vi "v2.61.vi"() -> ()   [LabVIEW 2018]
uses:
  <vilib>/DAQmx/read.llb/DAQmx Read (Analog 1D DBL NChan 1Samp).vi
  <extravilib>/ChannelInstances/High Speed Stream-c(a[.](c(dbl,dbl,dbl,dbl)),stamp,a[.](dbl),c(dbl,dbl,dbl,dbl,dbl,dbl,dbl))/_Read For Replicate.vi
  <extravilib>/ChannelInstances/High Speed Stream-c(a[.](c(dbl,dbl,dbl,dbl)),stamp,a[.](dbl),c(dbl,dbl,dbl,dbl,dbl,dbl,dbl))/Instantiate.vi
  <vilib>/Utility/file.llb/Write Delimited Spreadsheet (string).vi
  <extravilib>/ChannelInstances/High Speed Stream-c(a[.](c(dbl,dbl,dbl,dbl)),stamp,a[.](dbl),c(dbl,dbl,dbl,dbl,dbl,dbl,dbl))/)Channel.vi
  <extravilib>/ChannelInstances/High Speed Stream-c(a[.](c(dbl,dbl,dbl,dbl)),stamp,a[.](dbl),c(dbl,dbl,dbl,dbl,dbl,dbl,dbl))/Abort Signal/Init Signal.vi
  <vilib>/DAQmx/create/channels.llb/DAQmx Create Channel (AI-Temperature-Thermocouple).vi
  <vilib>/DAQmx/configure/timing.llb/DAQmx Timing (Sample Clock).vi
  <vilib>/DAQmx/miscellaneous.llb/DAQmx Fill In Error Info.vi
  <extravilib>/ChannelInstances/High Speed Stream-c(a[.](c(dbl,dbl,dbl,dbl)),stamp,a[.](dbl),c(dbl,dbl,dbl,dbl,dbl,dbl,dbl)).lvlib
panel:
  in  "file path (dialog if empty)":path
  out "Enum":T1(ring)
  in  "Start Recording?":bool
  in  "Stop Recording?":bool
  in  "Flowrate Control":dbl
  out "Status":T2(ring)
  in  "OK Button":bool
  in  "DAQ Properties":cluster{"Sample Rate":dbl}={"Sample Rate"=1.0} {"Sample Rate" min=1.0 max=10000.0 step=1.0}
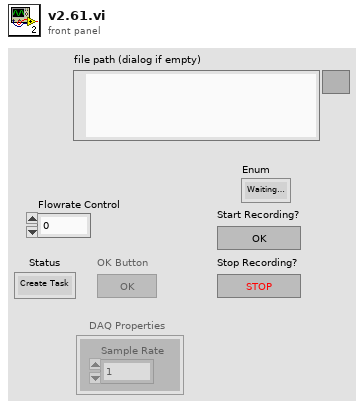
[diagram p1: front panel]
types:
  T1 = enum16{"Waiting to record", "Creating Spreadsheet", "Recording", "Finished Recording"}
  T2 = enum16{"Create Task", "Change Settings", "Check Settings", "Read Data", "End Task"}
  T3 = enum8{"Enabled", "Disabled", "Disabled and Grayed Out"}
  T4 = cluster{"Flowrate Data":cluster{"Line Number":dbl, "Temperature":dbl, "Pressure":dbl, "Flowrate":dbl}[], "Current Time":timestamp, "DAQmx Data":dbl[], "Rig Temperatures":cluster{"BRNR FC":dbl, "BRNR Nozzle":dbl, "Lance Tip":dbl, "Tube 2 Tmp":dbl, "Tube Tmp":dbl, "GA GAS Tmp":dbl, "Chamber External Temp":dbl}}
  T5 = cluster{"BRNR FC":dbl, "BRNR Nozzle":dbl, "Lance Tip":dbl, "Tube 2 Tmp":dbl, "Tube Tmp":dbl, "GA GAS Tmp":dbl, "Chamber External Temp":dbl}
  T6 = cluster{"Line Number":dbl, "Temperature":dbl, "Pressure":dbl, "Flowrate":dbl}[]
  T7 = typedef "High Speed Stream-c(a[.](c(dbl,dbl,dbl,dbl)),stamp,a[.](dbl),c(dbl,dbl,dbl,dbl,dbl,dbl,dbl)).lvlib/)Channel.ctl" = refnum<queue>
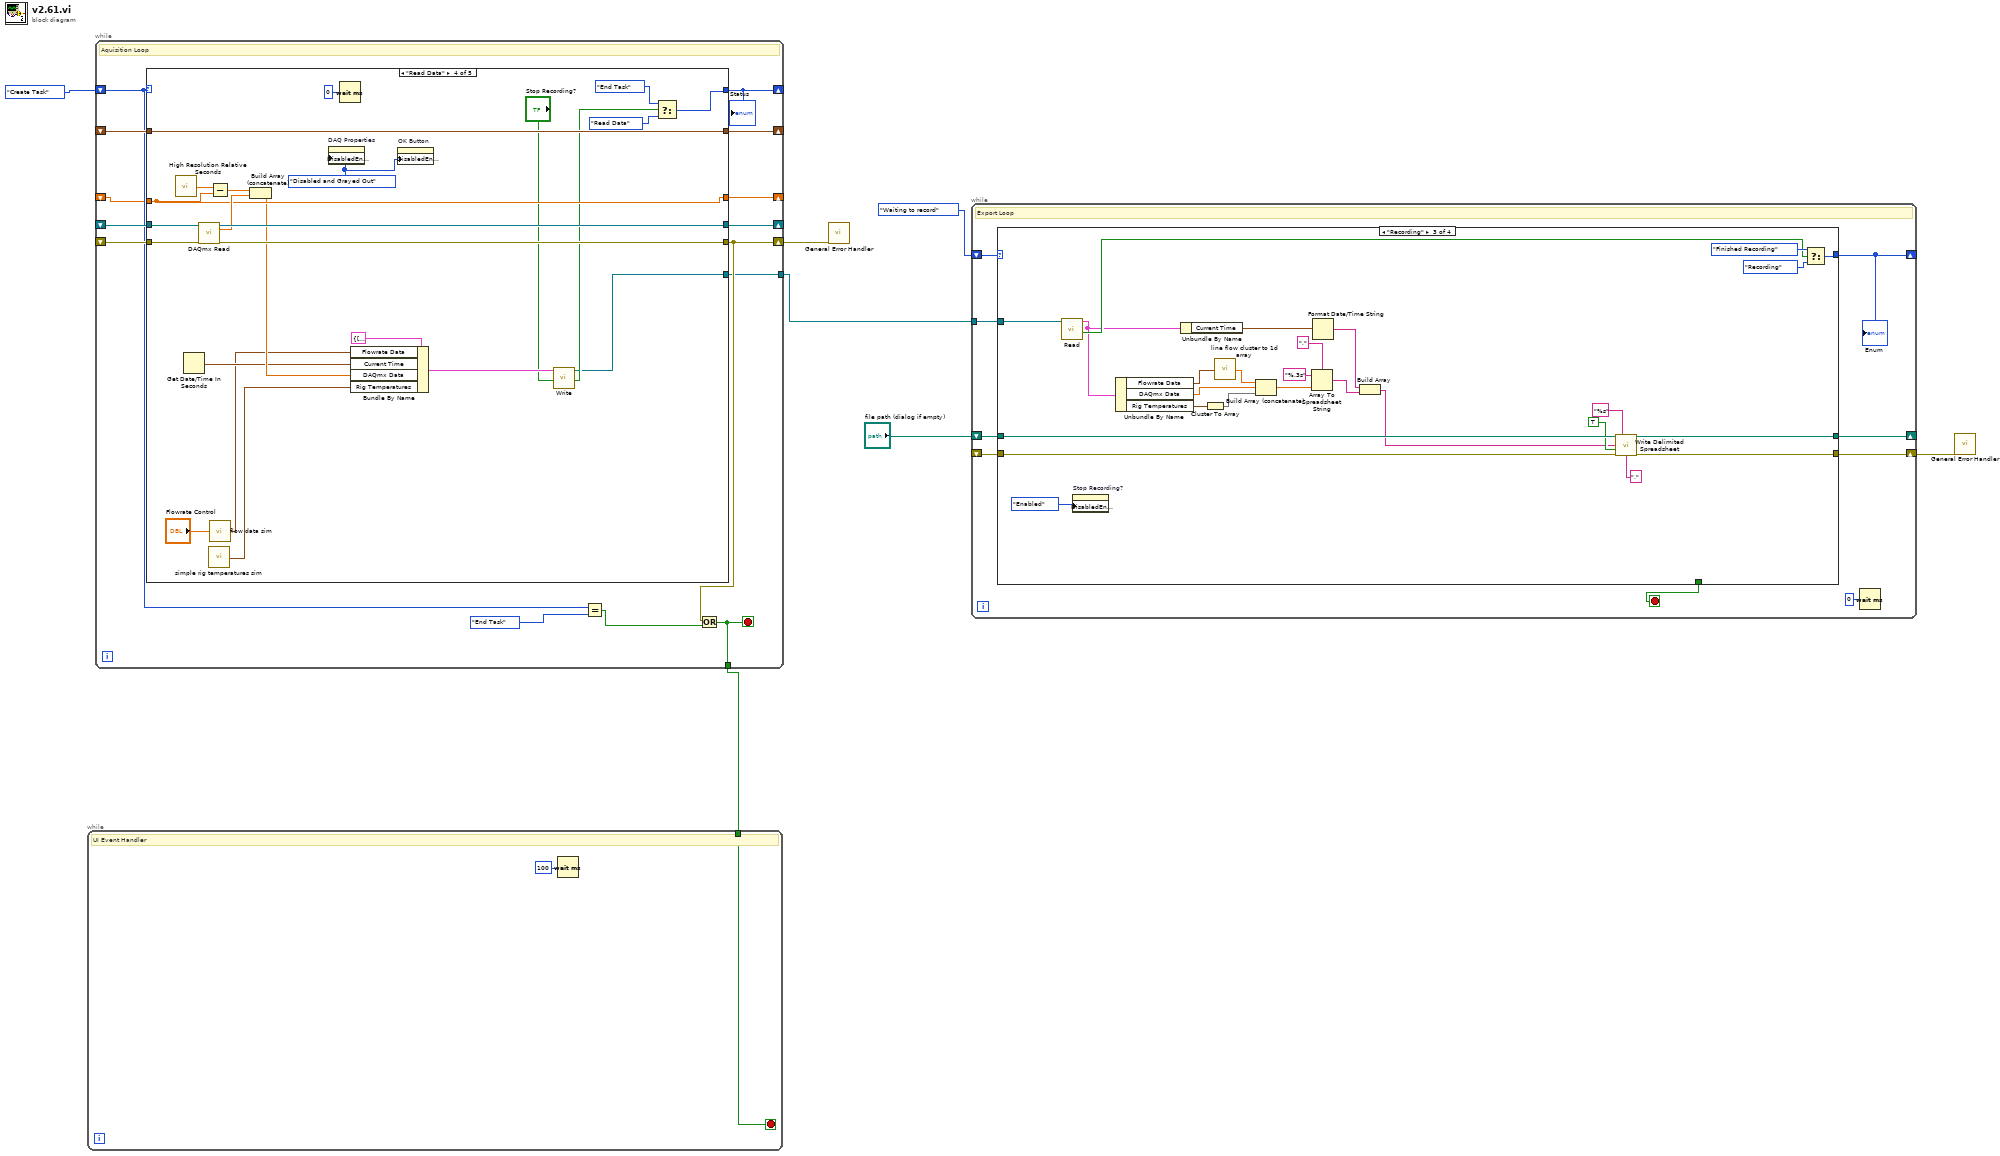
[diagram p0: block diagram]
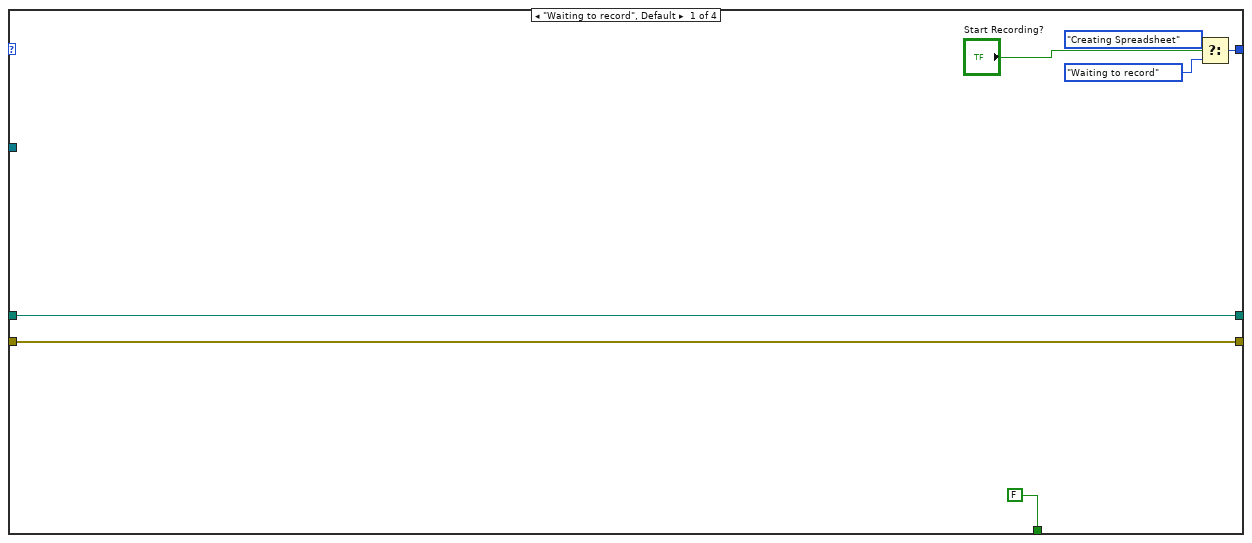
[diagram p2: hidden frame]
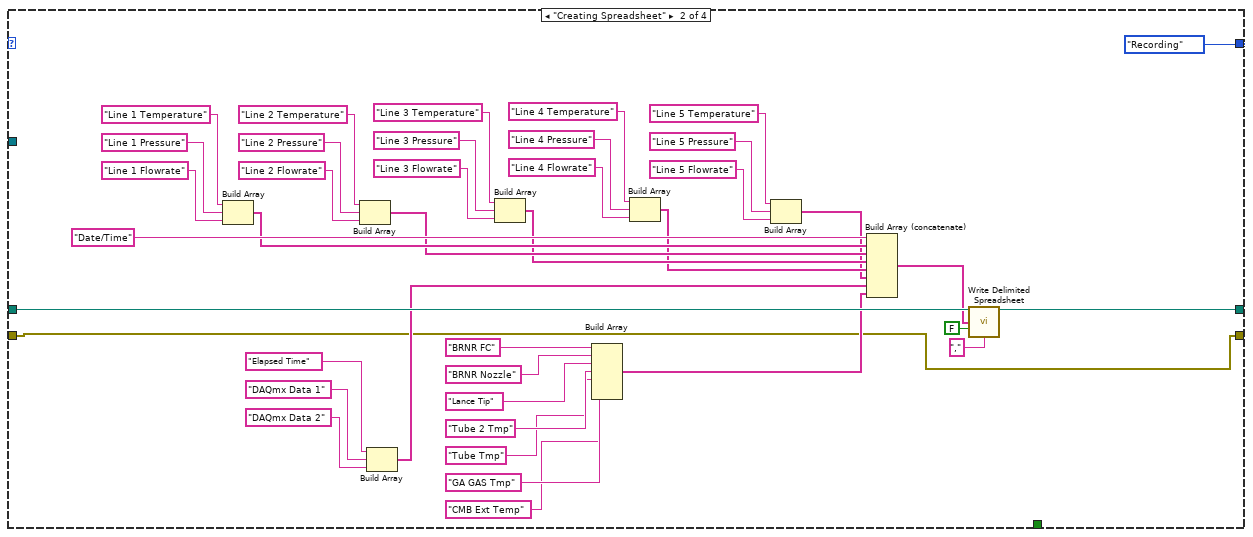
[diagram p3: hidden frame]
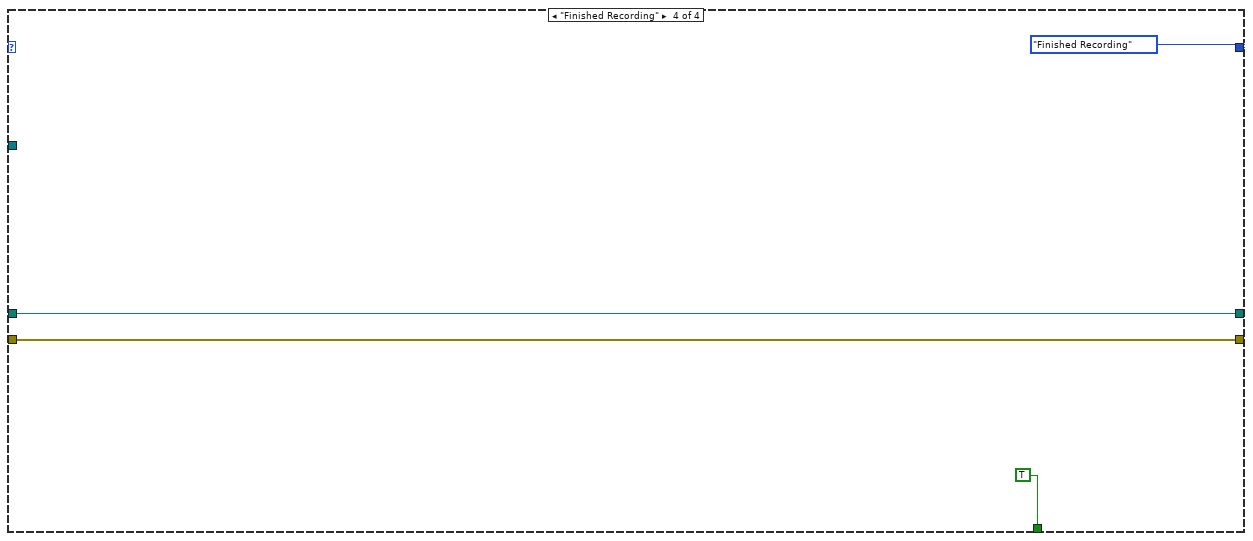
[diagram p4: hidden frame]
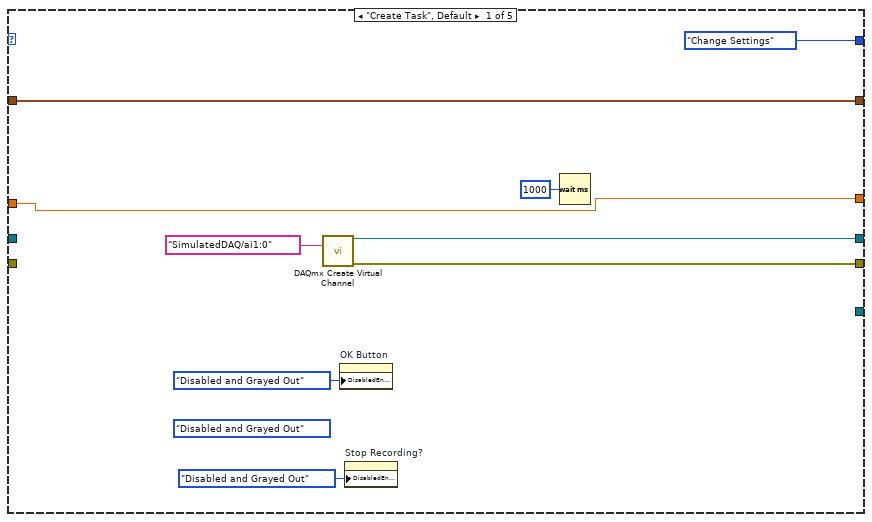
[diagram p5: hidden frame]
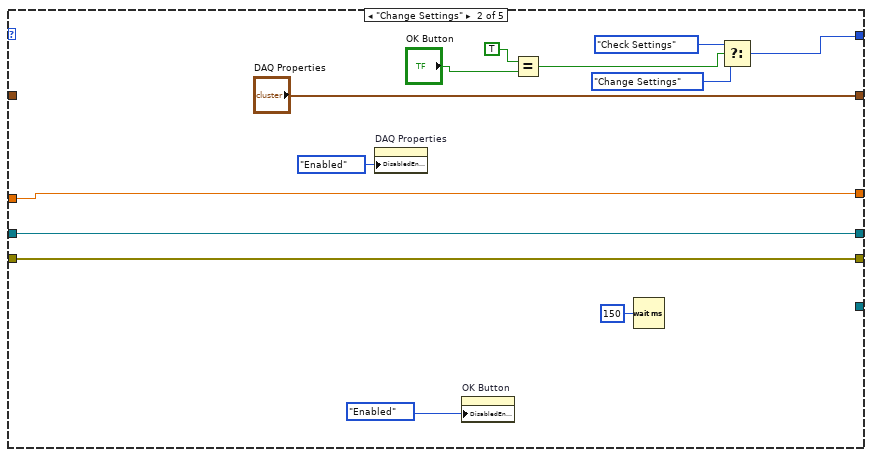
[diagram p6: hidden frame]
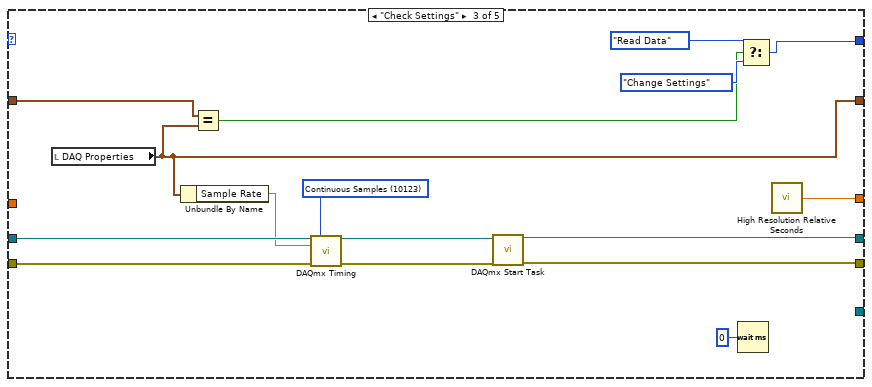
[diagram p7: hidden frame]
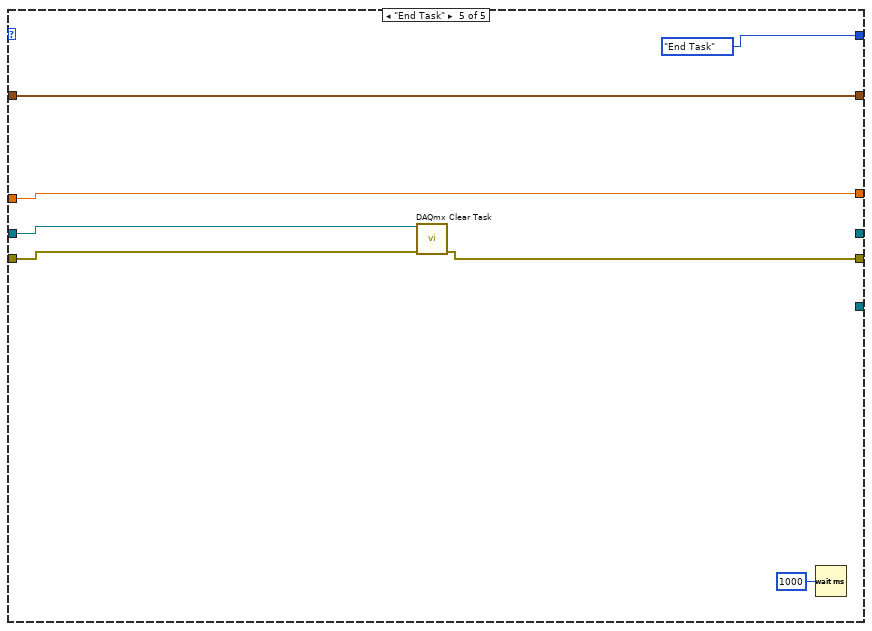
[diagram p8: hidden frame]
diagram:
  n1 = while {
    shift-right: [w16] -> _
    shift-left: T2."Create Task" -> [w12]
    shift-right: [w21] -> _
    shift-left: _ -> [w19]
    shift-right: [w15] -> w1
    shift-left: _ -> [w18]
    shift-right: [w20] -> _
    shift-left: _ -> [w17]
    shift-right: [w11] -> _
    shift-left: _ -> [w10]
    tunnel: [w9] -> w6
    tunnel: [w8] -> w4
    stop <- w9 stop-if-true
    # "Aquisition Loop"
    n2 = case shown="\"Read Data\"" w12 {
      tunnel: [w30 w43 w48 w80 _] -> w21
      tunnel: [w29 w42 w47 w79 w90] -> w15
      tunnel: [T2."Change Settings" w36 w55 w77 T2."End Task"] -> w16
      tunnel: [w26 "DAQ Properties" w51 w81 w89] -> w20
      tunnel: w19 -> [_ w43 w54 w83 w87]
      tunnel: w18 -> [_ w42 w53 w82 w86]
      tunnel: w17 -> [w26 _ w59 w81 w89]
      tunnel: [w24 w33 w44 w71 w85] -> w11
      tunnel: w10 -> [w24 w33 _ w71 w85]
      tunnel: [_ _ _ w60 _] -> w8
      frame "Create Task", Default {
        (unwired) T3."Disabled and Grayed Out" ("Disabled")
        n3 = call-poly <vilib>:"DAQmx Create Virtual Channel.vi"("physical channels"=tag "SimulatedDAQ/ai1:0") -> ("task out"=w30:refnum<k21>, "error out"=w29:errorcluster)  [unwired: 13 in]
        n4 = property on="OK Button" class="Bool"("DisabledEnum"=T3."Disabled and Grayed Out" ("Disabled")) -> ()  [unwired: 2 in, 2 out]
        n5 = property on="Stop Recording?" class="Bool"("DisabledEnum"=T3."Disabled and Grayed Out" ("Disabled")) -> ()  [unwired: 2 in, 2 out]
        n6 = Wait (ms)(milliseconds to wait=u32 1000) -> ()  [unwired: 1 out]
      }
      frame "Change Settings" {
        n7 = property on="DAQ Properties" class="Clust (strict)"("DisabledEnum"=T3."Enabled" ("Disabled")) -> ()  [unwired: 2 in, 2 out]
        n8 = property on="OK Button" class="Bool"("DisabledEnum"=T3."Enabled" ("Disabled")) -> ()  [unwired: 2 in, 2 out]
        n9 = Equal?(x=TRUE, y="OK Button") -> (x = y?=w38:bool)
        n10 = Wait (ms)(milliseconds to wait=u32 150) -> ()  [unwired: 1 out]
        n11 = Select(t=T2."Check Settings", s=w38, f=T2."Change Settings") -> (s? t:f=w36:T2)
      }
      frame "Check Settings" {
        w45 = 10123 items=["Finite Samples"=10178, "Continuous Samples"=10123, "Hardware Timed Single Point"=12522] ("sample mode")
        n12 = local read "DAQ Properties"() -> (w51:cluster{"Sample Rate":dbl})
        n13 = Unbundle By Name(w51) -> ("Sample Rate"=w52:dbl)
        n14 = Equal?(x=w59, y=w51) -> (x = y?=w46:bool)
        n15 = call-poly <vilib>:"DAQmx Timing.vi"("task/channels in"=w54, "sample mode"=w45, "rate"=w52, "error in"=w53) -> ("task out"=w50:refnum<k21>, "error out"=w49:errorcluster)  [unwired: 10 in]
        n16 = call <vilib>:"DAQmx Start Task.vi"("task/channels in"=w50, "error in"=w49) -> ("task out"=w48:refnum<k21>, "error out"=w47:errorcluster)  [unwired: 12 in]
        n17 = Wait (ms)(milliseconds to wait=u32 0) -> ()  [unwired: 1 out]
        n18 = Select(t=T2."Read Data", s=w46, f=T2."Change Settings") -> (s? t:f=w55:T2)
        n19 = call <vilib>:"High Resolution Relative Seconds.vi"() -> ("relative seconds"=w44:dbl)
      }
      frame "Read Data" {
        w69 = T3."Disabled and Grayed Out" ("Disabled")
        n20 = call <vilib>:"High Resolution Relative Seconds.vi"() -> ("relative seconds"=w74:dbl)
        n21 = Get Date/Time In Seconds() -> (seconds since 1Jan1904=w66:timestamp)
        n22 = call-poly <vilib>:"DAQmx Read.vi"("task/channels in"=w83, "error in"=w82) -> ("task out"=w80:refnum<k21>, "data"=w73:dbl[], "error out"=w79:errorcluster)  [unwired: 11 in]
        n23 = call "simple rig temperatures sim.vi"() -> ("Rig Temperatures"=w64:T5)
        n24 = call "flow data sim.vi"("Boondoggle Input"="Flowrate Control") -> ("Flowrate Data"=w65:T6)
        n25 = Subtract(x=w74, y=w71) -> (x-y=w72:dbl)
        n26 = Build Array (concatenate)(w72, w73) -> (w67:dbl[])
        n27 = property on="DAQ Properties" class="Clust (strict)"("DisabledEnum"=w69) -> ()  [unwired: 2 in, 2 out]
        n28 = Wait (ms)(milliseconds to wait=u32 0) -> ()  [unwired: 1 out]
        n29 = Bundle By Name(cluster=T4 {"Flowrate Data"=[{"Line Number"=1.0, "Temperature"=17.480721541683437, "Pressure"=24.0, "Flowrate"=0.0}, {"Line Number"=2.0, "Temperature"=21.850901927104296, "Pressure"=30.0, "Flowrate"=0.0}, {"Line Number"=3.0, "Temperature"=26.221082312525155, "Pressure"=36.0, "Flowrate"=0.0}, {"Line Number"=4.0, "Temperature"=30.591262697946018, "Pressure"=42.00000000000001, "Flowrate"=0.0}, {"Line Number"=5.0, "Temperature"=34.96144308336687, "Pressure"=48.0, "Flowrate"=0.0}], "Current Time"=timestamp(0 s since 1904-01-01), "DAQmx Data"=[], "Rig Temperatures"={"BRNR FC"=0.0, "BRNR Nozzle"=0.0, "Lance Tip"=0.0, "Tube 2 Tmp"=0.0, "Tube Tmp"=0.0, "GA GAS Tmp"=0.0, "Chamber External Temp"=0.0}}, "Flowrate Data"=w65, "Current Time"=w66, "DAQmx Data"=w67, "Rig Temperatures"=w64) -> (w63:T4)
        n30 = property on="OK Button" class="Bool"("DisabledEnum"=w69) -> ()  [unwired: 2 in, 2 out]
        n31 = call <extravilib>:"Write.vi"("last element? (F)"="Stop Recording?", "element"=w63) -> ("done?"=w61:bool, "channel"=w60:T7)  [unwired: 7 in, 1 out]
        n32 = Select(t=T2."End Task", s=w61, f=T2."Read Data") -> (s? t:f=w77:T2)
      }
      frame "End Task" {
        n33 = call <vilib>:"DAQmx Clear Task.vi"("task in"=w87, "error in"=w86) -> ("error out"=w90:errorcluster)  [unwired: 13 in]
        n34 = Wait (ms)(milliseconds to wait=u32 1000) -> ()  [unwired: 1 out]
      }
    }
    "Status" <- w16
    n35 = Equal?(x=w12, y=T2."End Task") -> (x = y?=w13:bool)
    n36 = Or(x=w15, y=w13) -> (x .or. y?=w9:bool)
  }
  n37 = while {
    tunnel: w6 -> [w91]
    stop <- w91 stop-if-true
    # "UI Event Handler"
    n38 = Wait (ms)(milliseconds to wait=u32 100) -> ()  [unwired: 1 out]
  }
  n39 = call <vilib>:"General Error Handler.vi"("error in (no error)"=w1) -> ()  [unwired: 10 in, 5 out]
  n40 = while {
    shift-right: [w100] -> _
    shift-left: T1."Waiting to record" -> [w99]
    tunnel: w4 -> [w97]
    shift-right: [w95] -> _
    shift-left: "file path (dialog if empty)" -> [w96]
    shift-right: [w94] -> w2
    shift-left: _ -> [w93]
    stop <- w98 stop-if-true
    # "Export Loop"
    n41 = case shown="\"Recording\"" w99 {
      tunnel: [w105 T1."Recording" w173 T1."Finished Recording"] -> w100
      tunnel: [FALSE _ _ TRUE] -> w98
      tunnel: w97 -> [_ _ w169 _]
      tunnel: w96 -> [w103 w127 w166 w176]
      tunnel: [w103 w126 w167 w176] -> w95
      tunnel: [w102 w109 w155 w175] -> w94
      tunnel: w93 -> [w102 w109 w154 w175]
      frame "Waiting to record", Default {
        n42 = Select(t=T1."Creating Spreadsheet", s="Start Recording?", f=T1."Waiting to record") -> (s? t:f=w105:T1)
      }
      frame "Creating Spreadsheet" {
        n43 = Build Array("Line 1 Temperature", "Line 1 Pressure", "Line 1 Flowrate") -> (w132:string[])
        n44 = Build Array("Line 2 Temperature", "Line 2 Pressure", "Line 2 Flowrate") -> (w131:string[])
        n45 = Build Array("Elapsed Time", "DAQmx Data 1", "DAQmx Data 2") -> (w119:string[])
        n46 = Build Array("Line 3 Temperature", "Line 3 Pressure", "Line 3 Flowrate") -> (w130:string[])
        n47 = Build Array("BRNR FC", "BRNR Nozzle", "Lance Tip", "Tube 2 Tmp", "Tube Tmp", "GA GAS Tmp", "CMB Ext Temp") -> (w111:string[])
        n48 = Build Array("Line 4 Temperature", "Line 4 Pressure", "Line 4 Flowrate") -> (w129:string[])
        n49 = Build Array("Line 5 Temperature", "Line 5 Pressure", "Line 5 Flowrate") -> (w120:string[])
        n50 = Build Array (concatenate)("Date/Time", w132, w131, w130, w129, w120, w119, w111) -> (w125:string[])
        n51 = call-poly <vilib>:"Write Delimited Spreadsheet.vi"("file path (dialog if empty)"=w127, "1D data"=w125, "append to file? (new file:F)"=FALSE, "delimiter (\\t)"="," ("delimiter (\\t)")) -> ("new file path (Not A Path if cancelled)"=w126:path)  [unwired: 10 in, 1 out]
      }
      frame "Recording" {
        n52 = call <extravilib>:"Read.vi"("channel"=w169) -> ("done?"=w168:bool, "element"=w163:T4)  [unwired: 6 in, 3 out]
        n53 = property on="Stop Recording?" class="Bool"("DisabledEnum"=T3."Enabled" ("Disabled")) -> ()  [unwired: 2 in, 2 out]
        n54 = Unbundle By Name(w163) -> ("Flowrate Data"=w164:T6, "DAQmx Data"=w160:dbl[], "Rig Temperatures"=w170:T5)
        n55 = Unbundle By Name(w163) -> ("Current Time"=w162:timestamp)
        n56 = Cluster To Array(cluster=w170) -> (array=w161:dbl[])
        n57 = call "line flow cluster to 1d array.vi"("Flowrate Data"=w164) -> ("Array"=w159:dbl[])
        n58 = Build Array (concatenate)(w159, w160, w161) -> (w158:dbl[])
        n59 = Array To Spreadsheet String(delimiter (Tab)=",", array=w158, 3:"%.3s" ("format string")) -> (spreadsheet string=w149:string)
        n60 = Format Date/Time String(seconds (now)=w162) -> (date/time string=w150:string)  [unwired: 2 in]
        n61 = Build Array(w150, w149) -> (w151:string[])
        n62 = call-poly <vilib>:"Write Delimited Spreadsheet.vi"("file path (dialog if empty)"=w166, "format (%s)"="%s", "1D data"=w151, "append to file? (new file:F)"=TRUE, "error in (no error)"=w154, "delimiter (\\t)"="," ("delimiter (\\t)")) -> ("new file path (Not A Path if cancelled)"=w167:path, "error out"=w155:errorcluster)  [unwired: 8 in]
        n63 = Select(t=T1."Finished Recording", s=w168, f=T1."Recording") -> (s? t:f=w173:T1)
      }
      frame "Finished Recording" {
      }
    }
    "Enum" <- w100
    n64 = Wait (ms)(milliseconds to wait=u32 0) -> ()  [unwired: 1 out]
  }
  n65 = call <vilib>:"General Error Handler.vi"("error in (no error)"=w2) -> ()  [unwired: 10 in, 5 out]
